vi "Listen.vi"(6 "clear_timeout_error (f)":bool, 7 "listener_port":u16, 8 "error in (no error)":errorcluster, 9 "service_name":string, 10 "net_address":string, 11 "Socket.TCP in":refnum<class "Socket.TCP.lvclass">) -> (0 "error out":errorcluster, 3 "Socket.TCP out":refnum<class "Socket.TCP.lvclass">)   [LabVIEW 2014, in "Socket.lvlib" / "Socket.TCP.lvclass"]
doc: "string net_address is the host address to listen on. If left blank, the listener will listen to all host addresses.\n\nu16 listener_port is the port number to listen on.\n\nstring service_name is optional. If specified, labview will register the service name and port in the NI service locator"
uses:
  Socket.TCP.lvclass
  Socket.Base/Socket.Base.lvclass/Socket.Base.ctl
  Socket.TCP.lvclass/Socket.TCP.ctl
  Socket.Base/Accessors/Read timeout.vi
  Accessors/Write listener_refnum.vi
  Accessors/Write tcp _refnum.vi
  Accessors/Write remote_address .vi
  Accessors/Write remote_port .vi
  Socket.Base/Accessors/Write connected.vi
panel:
  # "Optional IP address of the ethernet card to use. If left blank, the listener will listen to all ethernet interfaces"
  # "Port to listen on"
  # "Optional.  If used, then LabVIEW will register this name and port with the NI Service Locator"
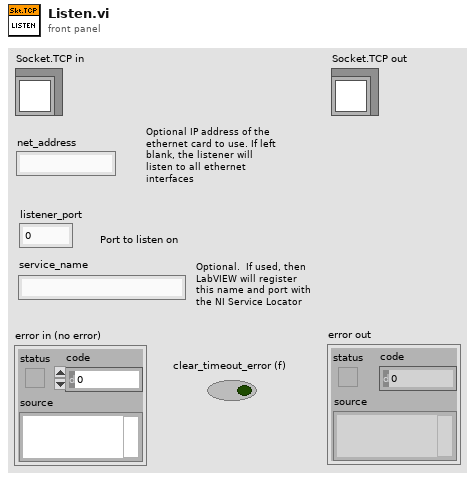
[diagram p1: front panel]
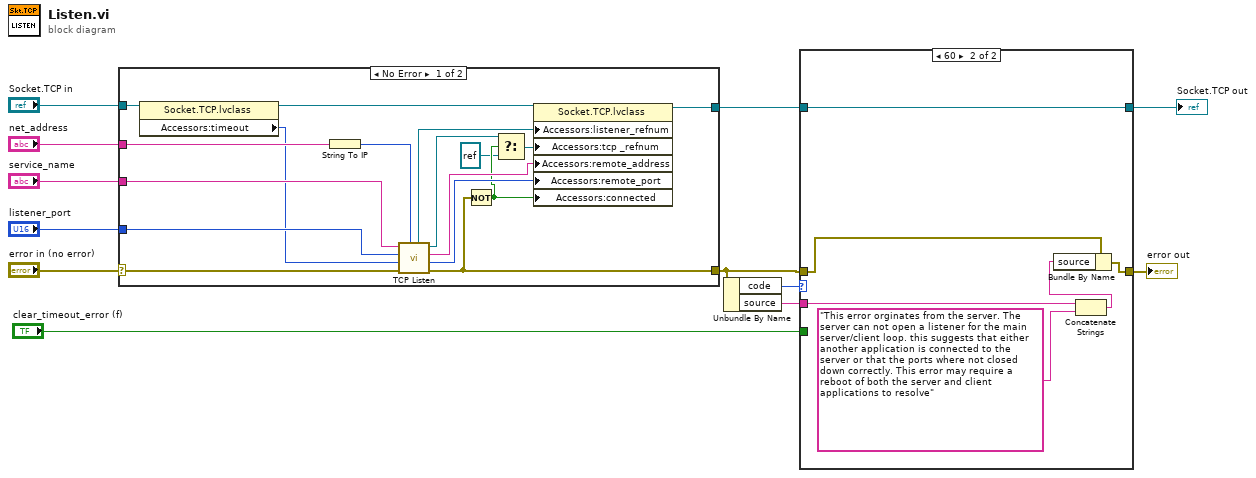
[diagram p0: block diagram]
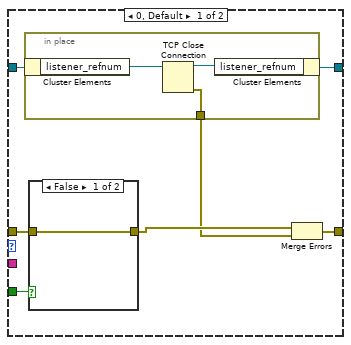
[diagram p2: hidden frame]
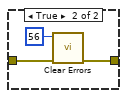
[diagram p3: hidden frame]
diagram:
  n1 = case shown="No Error" "error in (no error)" {
    selector: "error in (no error)" -> [w29 w31]
    tunnel: [w17 w31] -> w5
    tunnel: [w27 w30] -> w2
    tunnel: "Socket.TCP in" -> [w28 w30]
    tunnel: "net_address" -> [w25 _]
    tunnel: "service_name" -> [w24 _]
    tunnel: "listener_port" -> [w23 _]
    frame No Error {
      n2 = property class="Socket.TCP.lvclass"(reference=w28) -> (reference out=w19:refnum<class "Socket.TCP.lvclass">, "Accessors:timeout"=w18:i32)  [unwired: 1 in, 1 out]
      n3 = String To IP(1:w25) -> (0:w26:u32)
      n4 = call <vilib>:"TCP Listen.vi"("net address"=w26, "error in (no error)"=w29, "timeout ms (wait forever: -1)"=w18, "port"=w23, "service name"=w24) -> ("error out"=w17:errorcluster, "remote port"=w20:u16, "remote address"=w21:string, "connection ID"=w15:refnum<k5>, "listener ID"=w22:refnum<k5>)  [unwired: 2 in]
      n5 = Not(x=w17) -> (.not. x?=w14:bool)
      n6 = Select(t=w15, s=w14, f=refnum<k5> refnum) -> (s? t:f=w16:refnum<k5>)
      n7 = property class="Socket.TCP.lvclass"(reference=w19, "Accessors:listener_refnum"=w22, "Accessors:tcp _refnum"=w16, "Accessors:remote_address "=w21, "Accessors:remote_port "=w20, "Accessors:connected"=w14) -> (reference out=w27:refnum<class "Socket.TCP.lvclass">)  [unwired: 1 in, 1 out]
    }
    frame Error {
    }
  }
  n8 = Unbundle By Name(w5) -> ("code"=w7:i32, "source"=w6:string)
  n9 = case shown="60" w7 {
    tunnel: [w35 w48] -> w3
    tunnel: w6 -> [_ w51]
    tunnel: w5 -> [w38 w47]
    tunnel: "clear_timeout_error (f)" -> [w37 _]
    tunnel: w2 -> [w36 w46]
    tunnel: [w32 w46] -> w1
    frame 0, Default {
      n10 = in-place {
        in-place-border: [w39] -> w33
        n11 = in-place-cluster #1(w36) -> ("listener_refnum"=w41:refnum<k5>)
        n12 = TCP Close Connection(connection ID=w41) -> (connection ID out=w40:refnum<k5>, error out=w39:errorcluster)  [unwired: 2 in]
        n13 = in-place-cluster #1("listener_refnum"=w40) -> (w32:refnum<class "Socket.TCP.lvclass">)
      }
      n14 = case shown="False" w37 {
        tunnel: w38 -> [w42 w45]
        tunnel: [w42 w43] -> w34
        frame False {
        }
        frame True {
          n15 = call <vilib>:"Clear Errors.vi"("error in (no error)"=w45, "specific error code to clear (0: all)"=56) -> ("error out"=w43:errorcluster)  [unwired: 4 in, 1 out]
        }
      }
      n16 = Merge Errors(w34, w33) -> (w35:errorcluster)
    }
    frame 60 {
      n17 = Concatenate Strings(w51, "This error orginates from the server. The server can not open a listener for the main server/client loop. this suggests that either another application is connected to the server or that the ports where not closed down correctly. This error may require a reboot of both the server and client applications to resolve") -> (w49:string)
      n18 = Bundle By Name(cluster=w47, "source"=w49) -> (w48:errorcluster)
    }
  }
  "error out" <- w3
  "Socket.TCP out" <- w1
